vi "Stop_Watch.vi"() -> ()   [LabVIEW 2021]
doc: "This VI is a digital stop watch, which does the Same operations of normal Stop watches."
uses:
  Time_display.ctl
  Control_Cluster.ctl
panel:
  in  "Stop":bool
  out "Cluster 4":T1 {"ms" format="%#.2g"}
  in  "Cluster 3":T2
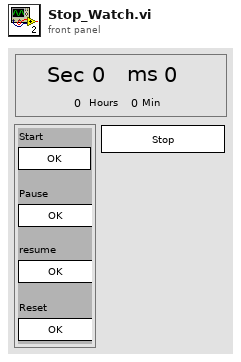
[diagram p1: front panel]
types:
  T1 = typedef "Time_display.ctl" = cluster{"Hours":i32, "Min":i32, "Sec":i32, "ms":i32}
  T2 = typedef "Control_Cluster.ctl" = cluster{"Start":bool, "Pause":bool, "resume":bool, "Reset":bool}
  T3 = typedef "LVDateTimeRec.ctl" = cluster{"fractional second":dbl, "second":i32, "minute":i32, "hour":i32, "day of month":i32, "month":i32, "year":i32, "day of week":i32, "day of year":i32, "DST":i32}
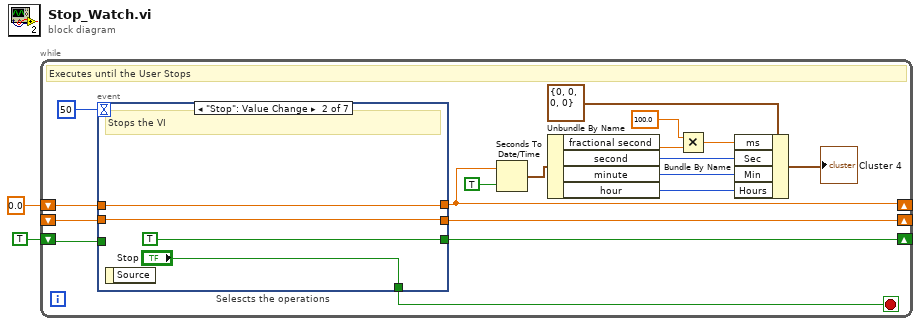
[diagram p0: block diagram]
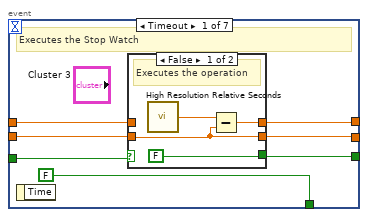
[diagram p2: hidden frame]
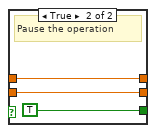
[diagram p3: hidden frame]
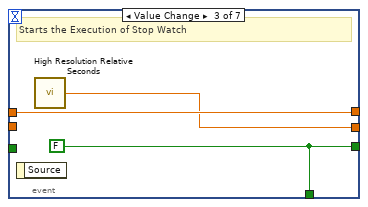
[diagram p4: hidden frame]
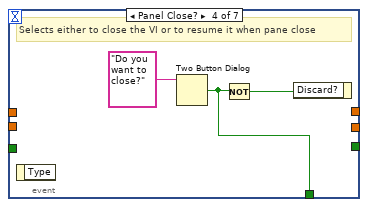
[diagram p5: hidden frame]
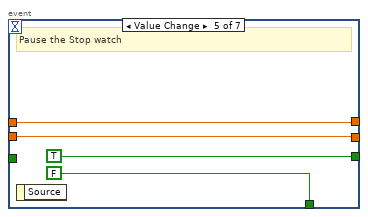
[diagram p6: hidden frame]
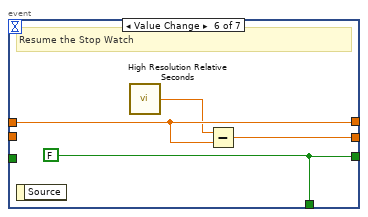
[diagram p7: hidden frame]
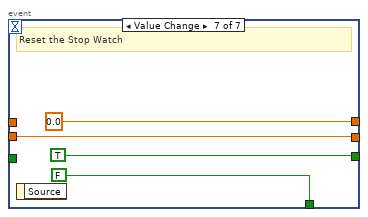
[diagram p8: hidden frame]
diagram:
  n1 = while {
    shift-right: [w18] -> _
    shift-left: TRUE -> [w19]
    shift-right: [w16] -> _
    shift-left: _ -> [w14]
    shift-right: [w7] -> _
    shift-left: 0.0 -> [w15]
    stop <- w17 stop-if-true
    # "Executes until the User Stops"
    n2 = event "Selescts the operations" shown="[1] \"Stop\": Value Change" {
      selector: _ -> [_ _ _ _ _ _ _]
      dyn-events: _ -> [_ _ _ _ _ _ _]
      timeout: 50 -> [_ _ _ _ _ _ _]
      tunnel: w19 -> [w27 _ _ _ _ _ _]
      tunnel: [w26 TRUE w39 _ TRUE w49 TRUE] -> w18
      tunnel: [FALSE "Stop" w39 w42 FALSE w49 FALSE] -> w17
      tunnel: w14 -> [w25 w37 _ _ w47 _ w55]
      tunnel: [w24 w37 w40 _ w47 w52 w55] -> w16
      tunnel: [w22 w36 w41 _ w48 w51 0.0] -> w7
      tunnel: w15 -> [w23 w36 w41 _ w48 w51 _]
      event Timeout {
        # "Executes the Stop Watch"
        n3 = event-data() -> ()  [unwired: 1 in, 1 out]
        n4 = case shown="False" w27 {
          tunnel: [FALSE TRUE] -> w26
          tunnel: w25 -> [w30 w33]
          tunnel: [w30 w33] -> w24
          tunnel: [w29 w32] -> w22
          tunnel: w23 -> [_ w32]
          frame False {
            # "Executes the operation"
            n5 = call <vilib>:"High Resolution Relative Seconds.vi"() -> ("relative seconds"=w28:dbl)
            n6 = Subtract(x=w28, y=w30) -> (x-y=w29:dbl)
          }
          frame True {
            # "Pause the operation"
          }
        }
      }
      event "Stop": Value Change {
        # "Stops the VI"
        n7 = event-data() -> ()  [unwired: 1 in, 1 out]
      }
      event Value Change {
        w39 = FALSE
        # "Starts the Execution of Stop Watch"
        n8 = event-data() -> ()  [unwired: 1 in, 1 out]
        n9 = call <vilib>:"High Resolution Relative Seconds.vi"() -> ("relative seconds"=w40:dbl)
      }
      event Panel Close? {
        # "Selects either to close the VI or to resume it when pane close"
        n10 = event-data() -> ()  [unwired: 1 in, 1 out]
        n11 = Two Button Dialog(message="Do you want to close?") -> (T button?=w42:bool)  [unwired: 2 in]
        n12 = Not(x=w42) -> (.not. x?=w43:bool)
        n13 = event-data("Discard?"=w43) -> ()  [unwired: 1 in, 1 out]
      }
      event Value Change {
        # "Pause the Stop watch"
        n14 = event-data() -> ()  [unwired: 1 in, 1 out]
      }
      event Value Change {
        w49 = FALSE
        # "Resume the Stop Watch"
        n15 = event-data() -> ()  [unwired: 1 in, 1 out]
        n16 = call <vilib>:"High Resolution Relative Seconds.vi"() -> ("relative seconds"=w50:dbl)
        n17 = Subtract(x=w50, y=w51) -> (x-y=w52:dbl)
      }
      event Value Change {
        # "Reset the Stop Watch"
        n18 = event-data() -> ()  [unwired: 1 in, 1 out]
      }
    }
    n19 = Seconds To Date/Time(time stamp (now)=w7, to UTC (F)=TRUE) -> (date time rec=w13:T3)
    n20 = Unbundle By Name(w13) -> ("fractional second"=w5:dbl, "second"=w10:i32, "minute"=w11:i32, "hour"=w12:i32)
    n21 = Multiply(x=100.0, y=w5) -> (x*y=w4:dbl)
    n22 = Bundle By Name(cluster=T1 {"Hours"=0, "Min"=0, "Sec"=0, "ms"=0} ("Cluster 3"), "ms"=w4, "Sec"=w10, "Min"=w11, "Hours"=w12) -> (→"Cluster 4":T1)
  }
